vi "ChangeLines(SubVI).vi"(8 "Error In":errorcluster, 10 "XYGraph Refnum":refnum<vi>, 11 "Arr Refnum":refnum<vi>) -> (0 "Error Out":errorcluster)   [LabVIEW 2018]
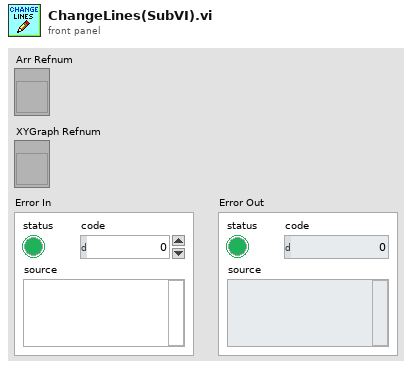
[diagram p1: front panel]
types:
  T1 = typedef "Line.ctl" = cluster{"Width":dbl, "Color":i64, "Array Oy":dbl[], "Array Ox":dbl[], "Name":string, "Plot Visible":T2}
  T2 = typedef "View.ctl" = bool
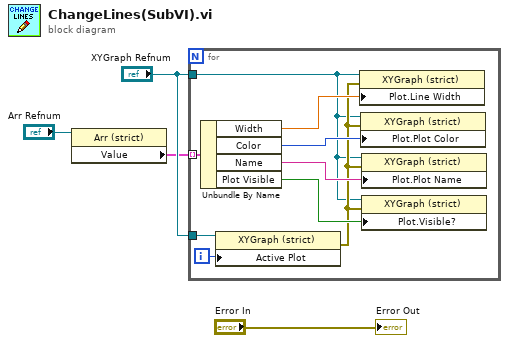
[diagram p0: block diagram]
diagram:
  n1 = property on="Property Node" class="Arr (strict)"(reference="Arr Refnum") -> ("Value"=w1:T1[])  [unwired: 1 in, 2 out]
  n2 = for {
    tunnel: w1 -> [w9] mode=indexing
    tunnel: "XYGraph Refnum" -> [w6]
    tunnel: "XYGraph Refnum" -> [w5]
    i -> [w8]
    n3 = Unbundle By Name(w9) -> ("Width"=w12:dbl, "Color"=w10:i64, "Name"=w13:string, "Plot Visible"=w11:T2)
    n4 = property on="Property Node" class="XYGraph (strict)"(reference=w5, "Active Plot"=w8) -> (error out=w7:errorcluster)  [unwired: 1 in, 1 out]
    n5 = property on="Property Node" class="XYGraph (strict)"(reference=w6, error in=w7, "Plot.Line Width"=w12) -> ()  [unwired: 2 out]
    n6 = property on="Property Node" class="XYGraph (strict)"(reference=w6, error in=w7, "Plot.Plot Color"=w10) -> ()  [unwired: 2 out]
    n7 = property on="Property Node" class="XYGraph (strict)"(reference=w6, error in=w7, "Plot.Plot Name"=w13) -> ()  [unwired: 2 out]
    n8 = property on="Property Node" class="XYGraph (strict)"(reference=w6, error in=w7, "Plot.Visible?"=w11) -> ()  [unwired: 2 out]
  }
  "Error Out" <- "Error In"
